vi "Array_to_Image.vi"(4 "PixelNum":i32, 6 "Image Properties":T2, 7 "Array":dbl[](array[numeric]), 8 "Channel":enum16{"Channel0", "Channel1"}(ring), 9 "Parameters":T1, 10 "Sum Num":u16, 11 "Color":i16) -> (3 "Array":u32[][](array[numeric]))   [LabVIEW 2016]
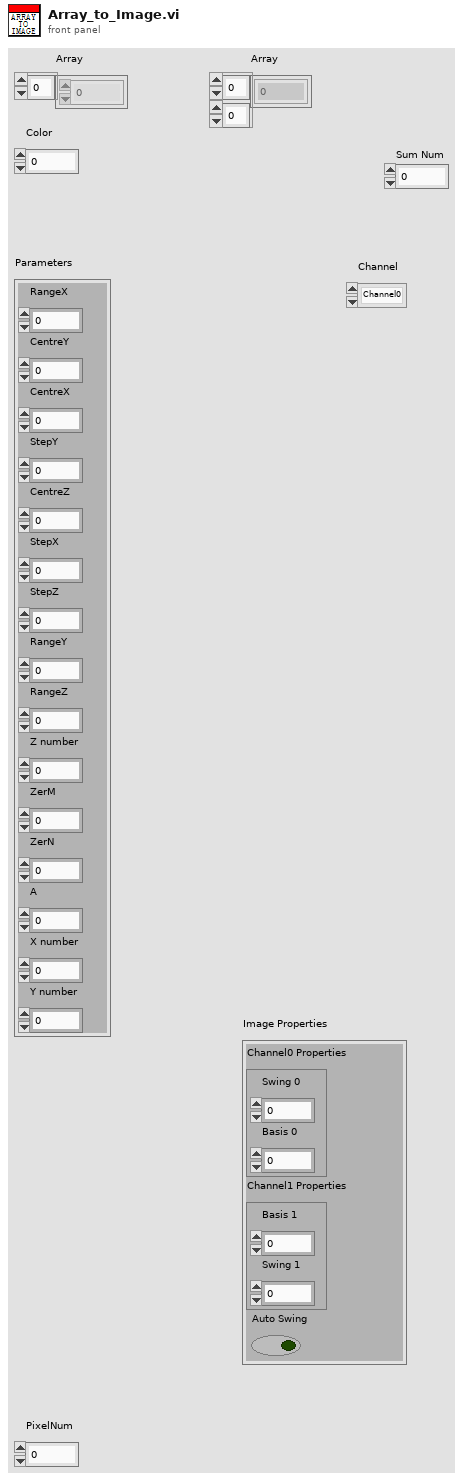
[diagram p1: front panel]
types:
  T1 = cluster{"RangeX":dbl, "CentreY":dbl, "CentreX":dbl, "StepY":dbl, "CentreZ":dbl, "StepX":dbl, "StepZ":dbl, "RangeY":dbl, "RangeZ":dbl, "Z number":i32, "ZerM":dbl, "ZerN":dbl, "A":dbl, "X number":i32, "Y number":i32}
  T2 = cluster{"Channel0 Properties":cluster{"Basis 0":dbl, "Swing 0":dbl}, "Channel1 Properties":cluster{"Basis 1":dbl, "Swing 1":dbl}, "Auto Swing":bool}
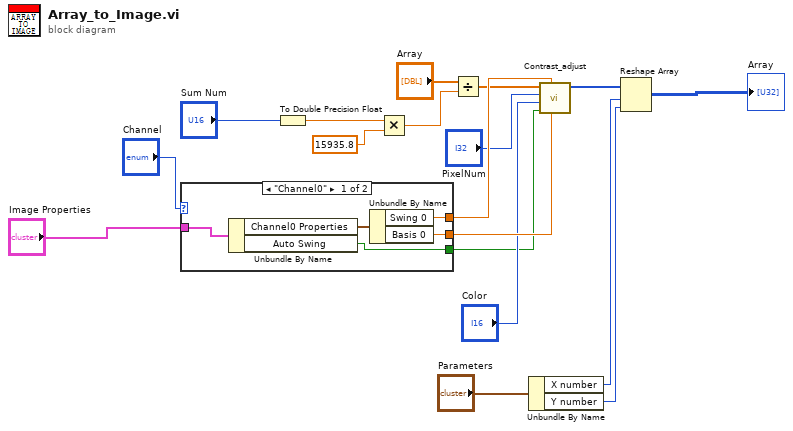
[diagram p0: block diagram]
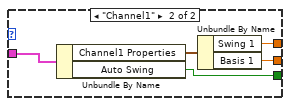
[diagram p2: hidden frame]
diagram:
  n1 = case shown="\"Channel0\"" "Channel" {
    tunnel: "Image Properties" -> [w23 w28]
    tunnel: [w21 w26] -> w17
    tunnel: [w20 w25] -> w18
    tunnel: [w19 w24] -> w2
    frame "Channel0" {
      n2 = Unbundle By Name(w23) -> ("Channel0 Properties"=w22:cluster{"Basis 0":dbl, "Swing 0":dbl}, "Auto Swing"=w19:bool)
      n3 = Unbundle By Name(w22) -> ("Swing 0"=w21:dbl, "Basis 0"=w20:dbl)
    }
    frame "Channel1" {
      n4 = Unbundle By Name(w28) -> ("Channel1 Properties"=w27:cluster{"Basis 1":dbl, "Swing 1":dbl}, "Auto Swing"=w24:bool)
      n5 = Unbundle By Name(w27) -> ("Swing 1"=w26:dbl, "Basis 1"=w25:dbl)
    }
  }
  n6 = To Double Precision Float(number="Sum Num") -> (double precision float=w3:dbl)
  n7 = Multiply(x=w3, y=15935.8) -> (x*y=w5:dbl)
  n8 = Divide(x="Array", y=w5) -> (x/y=w9:dbl[])
  n9 = Unbundle By Name("Parameters") -> ("X number"=w14:i32, "Y number"=w15:i32)
  n10 = call "Contrast_adjust.vi"("Basis"=w18, "Swing voltage"=w17, "Auto adjust"=w2, "Color"="Color", "Pixel number"="PixelNum", "Modulate date"=w9) -> ("Array"=w10:u32[])  [unwired: 5 in]
  n11 = Reshape Array(w10, w14, w15) -> (→"Array":u32[][])
